vi "Acquire Continuous Data.vi"(0 "VISA resource name":refnum<visa-resource-name>, 1 "Cluster Count (1)":dbl=1.0, 2 "Scan Interval (1)":dbl=1.0, 5 "Start Point (-120°)":dbl=-120.0, 7 "End Point (120°)":dbl=120.0, 9 "Number of Scans (0)":dbl, 11 "error in (no error)":errorcluster, 12 "Data Encoding Width (3 Byte)":u16(ring)=3 items=["2 Byte"=2, "3 Byte"=3], 13 "Enable Request Message (F:Disable)":bool) -> (4 "VISA resource name out":refnum<visa-resource-name>, 6 "Magnitude":dbl[](array[numeric]), 8 "Direction":dbl[](array[numeric]), 10 "Scan Ended?":bool, 14 "Number of Pending Scans":i32=1, 15 "error out":errorcluster)   [LabVIEW 2014, in "Hokuyo URG Series.lvlib"]
doc: "This VI takes four parameters (start point, end point, cluster count, number of scans) and returns two arrays which describe the magnitude and angle at which the data was acquired and number of pending scans. \n\nThe reference for the angles (in the Direction array) is the center of the device which is 0° with positive angles to the left of center and negative angles to the right.\n\nThe URG-04LX can take measurements in the range of -120° to 120° and has an \"operating range\" of -135° to 135°. \n\nCluster Count refers to the number of measurements which are clustered together. \n<b>Ex:</b>If the cluster count is 3 then the smallest of three measurements is returned.\n\nScan Interval refers to the number of scans to wait (no measurement is computed) after one measurement scan is performed.\n<b>Ex:</b>the scan interval should be less than 10.\n\nNumber of Scans refers to the total number of scans for which measurement is computed.\n<b>Ex:</b>A value of 0 means unlimited scans. The number of scans should be less than 100.\n\nThe Magnitude array is associated with the Direction array. \n<b>Ex:</b> If the information for the first measurement is desired, then the 0th index of each array is accessed and returns the magnitude and direction of the first measurement.\n\nScan Ended? specifies whether the scan is over or not.\n\nNumber of Pending Scans indicates how many more scans remain to be read, not including the current message. In the very last scan response message, the number of pending scans is set to 0, and when the number of scans is unlimited, the number of pending scans in all the scan response message is also 0.\n\nIf checksums are being used and the checksum fails, the data returned in the magnitude array will default to -1."
uses:
  Hokuyo URG Series.lvlib
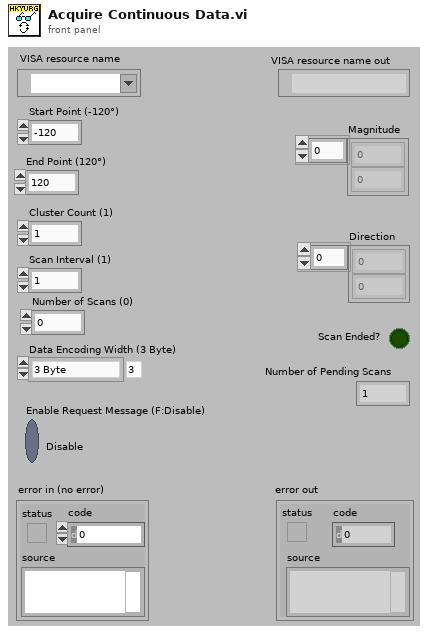
[diagram p1: front panel]
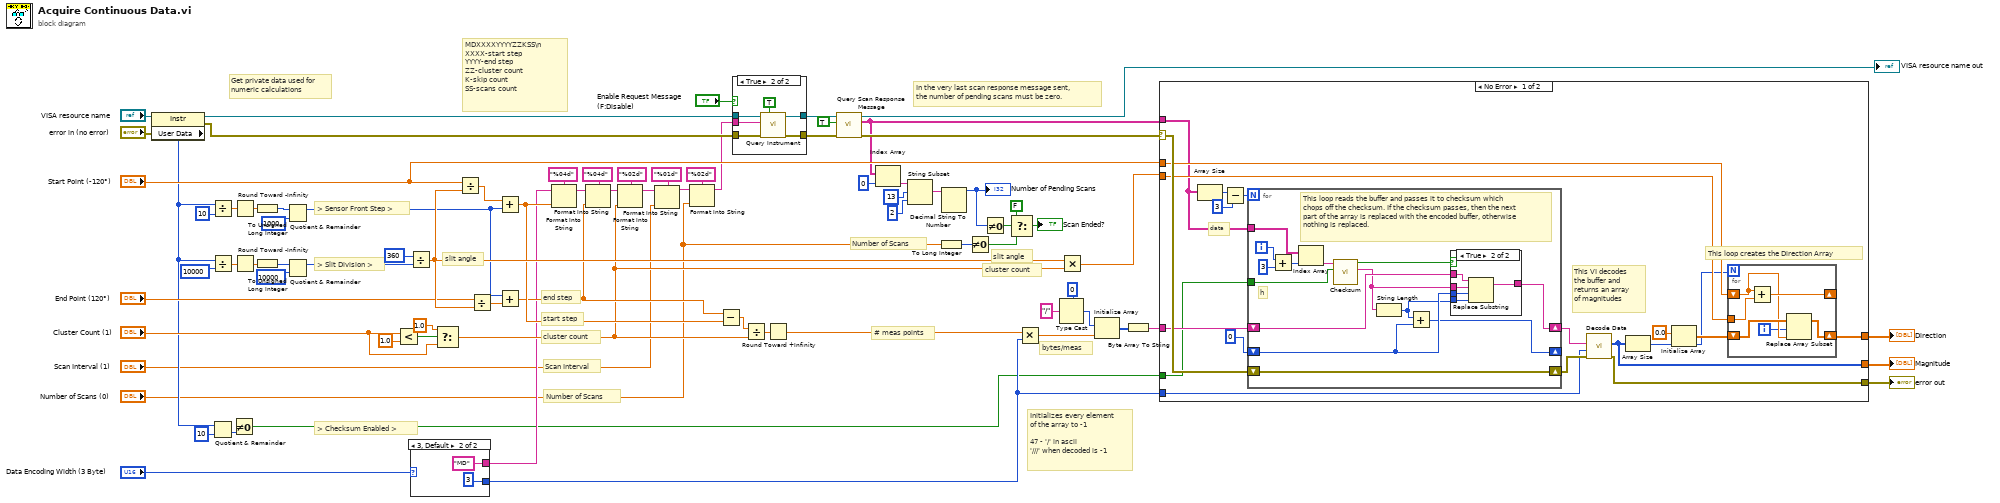
[diagram p0: block diagram]
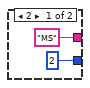
[diagram p3: hidden frame]
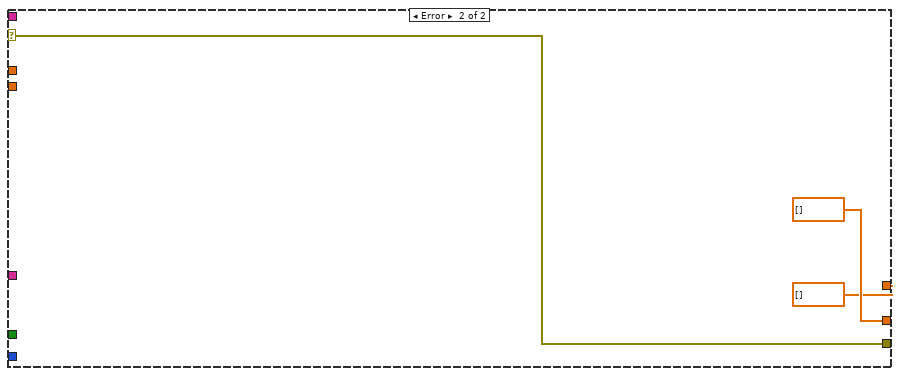
[diagram p5: hidden frame]
diagram:
  # "In the very last scan response message sent,\nthe number of pending scans must be zero."
  # "Number of Scans"
  # "cluster count"
  # "slit angle"
  # "Number of Scans"
  # "Scan Interval"
  # "Get private data used for numeric calculations"
  # "> Slit Division >"
  # "> Sensor Front Step >"
  # "> Checksum Enabled >"
  # "bytes/meas"
  # "# meas points"
  # "cluster count"
  # "start step"
  # "end step"
  # "slit angle"
  # "Initializes every element\nof the array to -1\n\n47 - '/' in ascii\n'///' when decoded is -1"
  # "MDXXXXYYYYZZKSS\\n\nXXXX-start step\nYYYY-end step\nZZ-cluster count\nK-skip count\nSS-scans count"
  n1 = property class="Instr"(reference="VISA resource name", error in="error in (no error)") -> (reference out=w32:refnum<visa-resource-name>, error out=w31:errorcluster, "User Data"=w34:u32)
  n2 = Divide(x=w34, y=u32 10) -> (x/y=w47:dbl)
  n3 = Divide(x=w34, y=u32 10000) -> (x/y=w41:dbl)
  n4 = Quotient & Remainder(x=w34, y=u32 10) -> (x-y*floor(x/y)=w48:u32)  [unwired: 1 out]
  n5 = Not Equal To 0?(x=w48) -> (x != 0?=w12:bool)
  n6 = Round Toward -Infinity(1:w47) -> (0:w43:dbl)
  n7 = Round Toward -Infinity(1:w41) -> (0:w40:dbl)
  n8 = To Unsigned Long Integer(number=w43) -> (unsigned 32bit integer=w46:u32)
  n9 = To Unsigned Long Integer(number=w40) -> (unsigned 32bit integer=w39:u32)
  n10 = Quotient & Remainder(x=w46, y=u32 1000) -> (x-y*floor(x/y)=w45:u32)  [unwired: 1 out]
  n11 = Quotient & Remainder(x=w39, y=u32 10000) -> (x-y*floor(x/y)=w37:u32)  [unwired: 1 out]
  n12 = Less?(x="Cluster Count (1)", y=1.0) -> (x < y?=w64:bool)
  n13 = Divide(x=u32 360 ("y"), y=w37) -> (x/y=w60:dbl)
  n14 = case shown="3, Default" "Data Encoding Width (3 Byte)" {
    tunnel: ["MS" ("initial string") "MD" ("initial string")] -> w29
    tunnel: [2 ("byte encoding width") 3 ("byte encoding width")] -> w28
    frame 2 {
    }
    frame 3, Default {
    }
  }
  n15 = Select(t=1.0, s=w64, f="Cluster Count (1)") -> (s? t:f=w52:dbl)
  n16 = Divide(x="Start Point (-120°)", y=w60) -> (x/y=w58:dbl)
  n17 = Divide(x="End Point (120°)", y=w60) -> (x/y=w55:dbl)
  n18 = Add(x=w58, y=w45) -> (x+y=w57:dbl)
  n19 = Add(x=w45, y=w55) -> (x+y=w54:dbl)
  n20 = Format Into String(format string="%04d", initial string=w29, w57) -> (resulting string=w74:string)  [unwired: 1 in, 1 out]
  n21 = Format Into String(format string="%04d", initial string=w74, w54) -> (resulting string=w72:string)  [unwired: 1 in, 1 out]
  n22 = Format Into String(format string="%02d", initial string=w72, w52) -> (resulting string=w23:string)  [unwired: 1 in, 1 out]
  n23 = Format Into String(format string="%01d", initial string=w23, "Scan Interval (1)") -> (resulting string=w25:string)  [unwired: 1 in, 1 out]
  n24 = Format Into String(format string="%02d", initial string=w25, "Number of Scans (0)") -> (resulting string=w22:string)  [unwired: 1 in, 1 out]
  n25 = Subtract(x=w54, y=w57) -> (x-y=w69:dbl)
  n26 = case shown="True" "Enable Request Message (F:Disable)" {
    tunnel: w32 -> [w85 w91]
    tunnel: w31 -> [w84 w90]
    tunnel: w22 -> [_ w88]
    tunnel: [w84 w87] -> w20
    tunnel: [w85 w86] -> w19
    frame False {
    }
    frame True {
      n27 = call "Query Instrument.vi"("Error Query (Enabled)"=TRUE, "error in"=w90, "Command"=w88, "VISA Resource Name"=w91) -> ("error out"=w87:errorcluster, "VISA Resource Name Out"=w86:refnum<visa-resource-name>)  [unwired: 5 in, 1 out]
    }
  }
  n28 = Divide(x=w69, y=w52) -> (x/y=w70:dbl)
  n29 = Round Toward +Infinity(x=w70) -> (ceil(x): smallest int >= x=w67:dbl)
  n30 = call "Query Scan Response Message.vi"("error in"=w20, "Error Query (Enabled)"=TRUE, "VISA resource name"=w19) -> ("error out"=w18:errorcluster, "Response Strings"=w14:string[], "VISA resource name out"=→"VISA resource name out":refnum<visa-resource-name>)  [unwired: 6 in]
  n31 = Index Array(array=w14, index=0) -> (element=w11:string)
  n32 = String Subset(string=w11, offset (0)=13, length (rest)=2 ("length (rest)")) -> (substring=w7:string)
  n33 = To Long Integer(number="Number of Scans (0)") -> (32bit integer=w3:i32)
  n34 = Decimal String To Number(string=w7) -> (number=w1:i32)  [unwired: 2 in, 1 out]
  "Number of Pending Scans" <- w1
  n35 = Not Equal To 0?(x=w3) -> (x != 0?=w4:bool)
  n36 = Not Equal To 0?(x=w1) -> (x != 0?=w6:bool)
  n37 = Select(t=FALSE, s=w6, f=w4) -> (s? t:f=→"Scan Ended?":bool)
  n38 = Multiply(x=w67, y=w28) -> (x*y=w66:dbl)
  n39 = Type Cast(type=u8 0, x="/") -> (*(type *) &x=w49:u8)
  n40 = Multiply(x=w60, y=w52) -> (x*y=w71:dbl)
  n41 = Initialize Array(w49, w66) -> (w68:u8[])
  n42 = Byte Array To String(unsigned byte array=w68) -> (string=w62:string)
  n43 = case shown="No Error" w18 {
    selector: w18 -> [w110 w139]
    tunnel: [w98 w139] -> w77
    tunnel: "Start Point (-120°)" -> [w109 _]
    tunnel: w71 -> [w108 _]
    tunnel: [w103 dbl[] []] -> w79
    tunnel: [w107 dbl[] []] -> w78
    tunnel: w62 -> [w106 _]
    tunnel: w12 -> [w97 _]
    tunnel: w14 -> [w92 _]
    tunnel: w28 -> [w93 _]
    frame No Error {
      # "data"
      # "This loop creates the Direction Array"
      # "This VI decodes the buffer and returns an array of magnitudes"
      n44 = Array Size(array=w92) -> (size(s)=w96:i32)
      n45 = Subtract(x=w96, y=3) -> (x-y=w95:i32)
      n46 = for {
        N: w95 -> [_]
        shift-right: [w111] -> w104
        shift-left: w110 -> [w111]
        shift-right: [w124] -> w105
        shift-left: w106 -> [w123]
        shift-right: [w121] -> _
        shift-left: 0 -> [w122]
        tunnel: w97 -> [w119]
        tunnel: w92 -> [w118]
        i -> [w116]
        # "h"
        # "This loop reads the buffer and passes it to checksum which chops off the checksum. If the checksum passes, then the next part of the array is replaced with the encoded buffer, otherwise nothing is replaced."
        n47 = Add(x=w116, y=3) -> (x+y=w117:i32)
        n48 = Index Array(array=w118, index=w117) -> (element=w114:string)
        n49 = call "Checksum.vi"("Checksum (Off)"=w119, "Input"=w114) -> ("Data Buffer"=w113:string, "Checksum Pass?"=w120:bool)  [unwired: 8 out]
        n50 = String Length(string=w113) -> (length=w112:i32)
        n51 = Add(x=w112, y=w122) -> (x+y=w121:i32)
        n52 = case shown="True" w120 {
          tunnel: [w125 w126] -> w124
          tunnel: w123 -> [w125 w130]
          tunnel: w113 -> [_ w129]
          tunnel: w122 -> [_ w128]
          tunnel: w112 -> [_ w127]
          frame False {
          }
          frame True {
            n53 = Replace Substring(2:w127, 3:w128, 4:w129, 5:w130) -> (1:w126:string)  [unwired: 1 out]
          }
        }
      }
      n54 = call "Decode Data.vi"("error in (no error)"=w104, "n character encoding"=w93, "Input Buffer"=w105) -> ("error out"=w98:errorcluster, "Decoded Measurements"=w103:i32[])  [unwired: 2 in, 5 out]
      n55 = Array Size(array=w103) -> (size(s)=w100:i32)
      n56 = Initialize Array(0.0 ("element"), w100) -> (w101:dbl[])
      n57 = for {
        N: w100 -> [_]
        shift-right: [w135] -> _
        shift-left: w109 -> [w132]
        tunnel: w108 -> [w136]
        shift-right: [w133] -> w107
        shift-left: w101 -> [w134]
        i -> [w131]
        n58 = Add(x=w132, y=w136) -> (x+y=w135:dbl)
        n59 = Replace Array Subset(array=w134, new element=w132, index=w131) -> (w133:dbl[])
      }
    }
    frame Error {
    }
  }
  "Magnitude" <- w79
  "Direction" <- w78
  "error out" <- w77
